vi "MPS_global_variables.vi"() -> ()   [LabVIEW 2021]
panel:
  in  "N Harmonics":dbl=40.0
  in  "Tx TF File":string(combo)="TxTF_IMonNotch-Inv.mat"
  in  "Rx TF File":string(combo)="MPS_RxTF_NotchUpdatedG000.mat"
  in  "TxIMon range":dbl=1.0
  in  "Fan Control Line":tag="H1/port0/line6"
  in  "mT/Bias Amp":dbl=9.36
  in  "mT/Drive Amp":dbl=0.45533
  in  "Drive IMon\nRef Freq":dbl=23809.0
  in  "Volts Per Amp\nBias":dbl=0.0375
  in  "Volts Per Amp\nDrive":dbl=0.0075657
  out "mT/BMon Volt":dbl=145.2509167046147
  in  "Analog Input Start Trig":tag="/H1/ai/StartTrigger"
  in  "Bias Output Chan.":tag="H2/ao1"
  in  "Drive Output Chan.":tag="H2/ao0"
  in  "B-Mon chan. mode":i32(ring)=10106 items=["Default"=-1, "RSE"=10083, "NRSE"=10078, "Differential"=10106, "Pseudodifferential"=12529]
  in  "Rx chan. mode":i32(ring)=10106 items=["Default"=-1, "RSE"=10083, "NRSE"=10078, "Differential"=10106, "Pseudodifferential"=12529]
  in  "B-Mon sense channel":tag="H1/ai6"
  in  "Drive I-Mon chan. mode":i32(ring)=10106 items=["Default"=-1, "RSE"=10083, "NRSE"=10078, "Differential"=10106, "Pseudodifferential"=12529]
  in  "Bias I-Mon chan. mode":i32(ring)=10083 items=["Default"=-1, "RSE"=10083, "NRSE"=10078, "Differential"=10106, "Pseudodifferential"=12529]
  in  "Rx channel":tag="H1/ai7"
  in  "Drive current meas. channel":tag="H1/ai4"
  in  "Bias I-Mon channel":tag="H1/ai5"
  in  "TxRx_Params":T1={"sample rate"=2000000.0, "Tx freq"=23809.52380952381, "Tx amp"=1.0, "Tx cycles\nSpectroscopy"=2000.0, "Bias amp"=2.65, "Bias freq"=11.904761904761905, "Receive range"=5.0, "Bias Periods\nMagnetometry"=2.0, "Tx Freq Division Factor"=84.0, "Drive Periods per Bias"=2000.0, "TX harmonics"=[47619.04761904762, 71428.57142857142, 95238.09523809524, 119047.61904761905, 142857.14285714284, 166666.66666666666, 190476.19047619047, 214285.7142857143, 238095.2380952381, 261904.7619047619, 285714.2857142857, 309523.8095238095, 333333.3333333333, 357142.85714285716, 380952.38095238095, 404761.90476190473, 428571.4285714286, 452380.95238095237]} {"TX harmonics" format="%#_4p"}
  in  "Device Name":tag="DAQ2"
  # "DAQ settings"
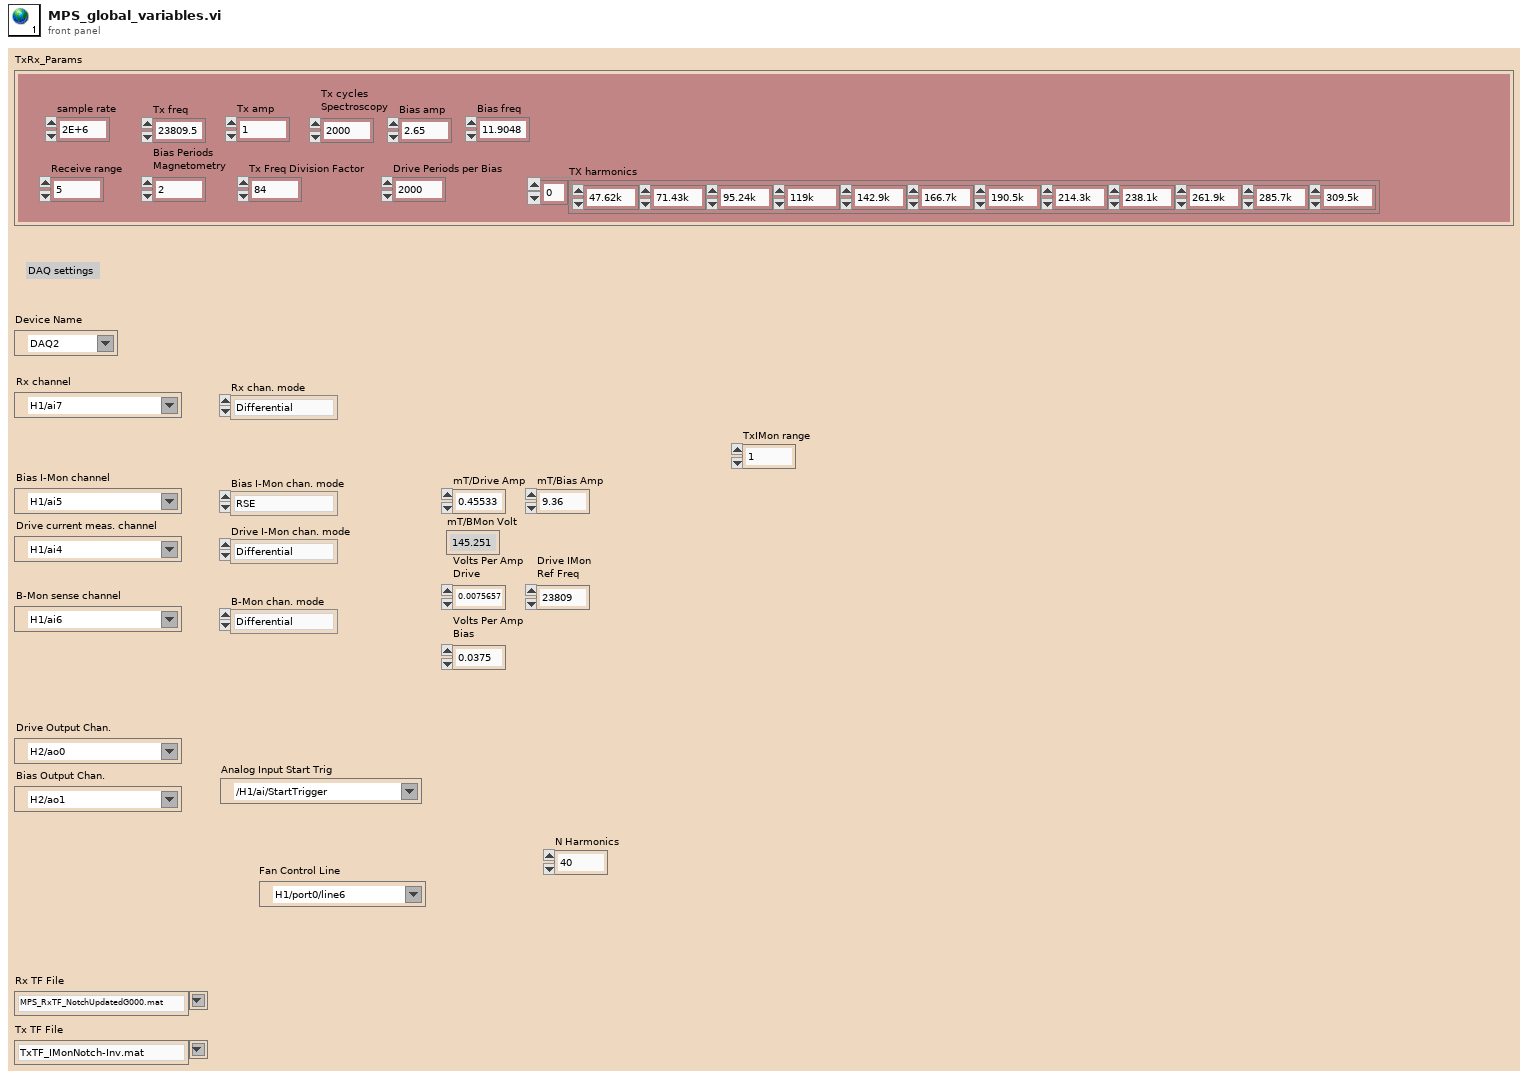
[diagram p1: front panel]
types:
  T1 = cluster{"sample rate":dbl, "Tx freq":dbl, "Tx amp":dbl, "Tx cycles\nSpectroscopy":dbl, "Bias amp":dbl, "Bias freq":dbl, "Receive range":dbl, "Bias Periods\nMagnetometry":dbl, "Tx Freq Division Factor":dbl, "Drive Periods per Bias":dbl, "TX harmonics":dbl[]}
diagram:
